vi "AV Write Single.vi"(8 "error in":errorcluster, 9 "Channel Index":i32=1, 10 "Actual Value":dbl, 11 "Power Actual Value in":refnum<class "Power Actual Value.lvclass">) -> (0 "error out":errorcluster, 3 "Power Actual Value out":refnum<class "Power Actual Value.lvclass">)   [LabVIEW 2023, in "Power Actual Value.lvclass"]
uses:
  Power Actual Value.lvclass
  Power Actual Value.lvclass/Power Actual Value.ctl
  Parents/Actual Value/Actual Value.lvclass
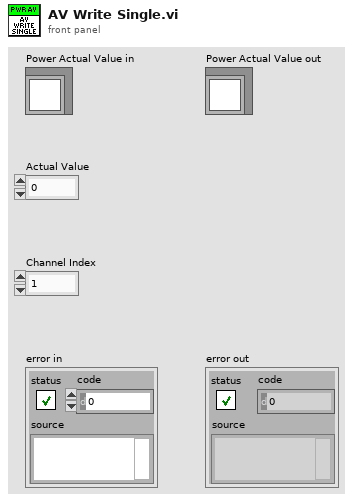
[diagram p1: front panel]
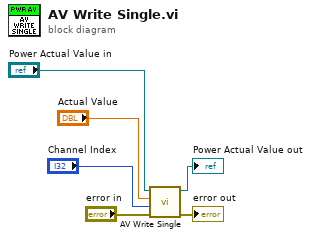
[diagram p0: block diagram]
diagram:
  n1 = call-parent "AV Write Single.vi"("error in"="error in", "Channel Index"="Channel Index", "Actual Value"="Actual Value", "Actual Value in"="Power Actual Value in") -> ("error out"=→"error out":errorcluster, "Actual Value out"=→"Power Actual Value out":refnum<class "Power Actual Value.lvclass">)  [unwired: 6 in]
